vi "KillProcessName.vi"(3 "error in (no error)":errorcluster, 5 "Process Name":string="USBSTOR\\DISK*") -> (0 "error out":errorcluster, 1 "Success":bool=TRUE, 2 "Command Output":string="USBSTOR\\DISK&VEN_KINGSTON&PROD_DT_101_G2&REV_PMAP\\001CC0EC34C7EB8145E3016C&0: Kingston DT 101 G2 USB Device\r\nUSBSTOR\\DISK&VEN_SANDISK&PROD_CRUZER&REV_1.00\\20043411200CF763653E&0: SanDisk Cruzer USB Device\r\n2 matching device(s) found.\r\n")   [LabVIEW 2013]
doc: "This VI can restart a usb device or disconnect first then scan for new device."
panel:
  out "return code":i32
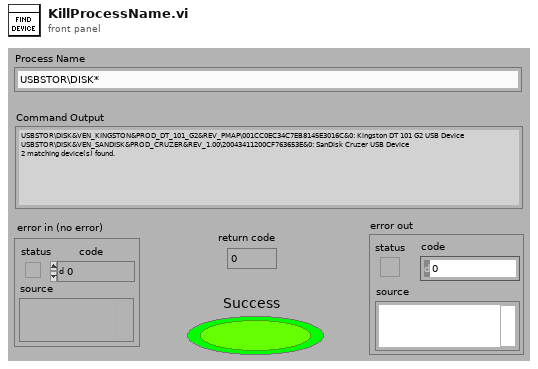
[diagram p1: front panel]
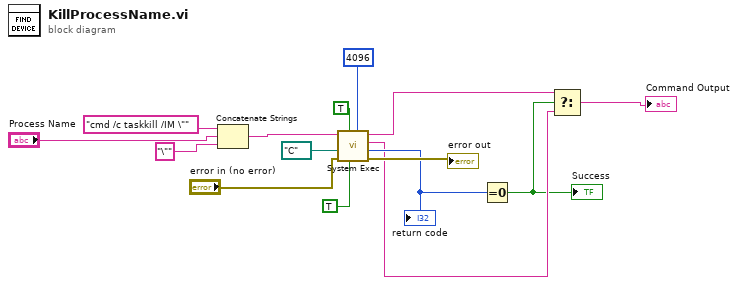
[diagram p0: block diagram]
diagram:
  n1 = Concatenate Strings("cmd /c taskkill /IM \"" ("command line"), "Process Name", "\"" ("string")) -> (w11:string)
  n2 = call <vilib>:"System Exec.vi"("expected output size  (4096)"=u32 4096, "run minimized? (F)"=TRUE, "wait until completion? (T)"=TRUE, "error in (no error)"="error in (no error)", "working directory"=path "C:/", "command line"=w11) -> ("error out"=→"error out":errorcluster, "return code"=w5:i32, "standard error"=w3:string, "standard output"=w4:string)  [unwired: 2 in]
  "return code" <- w5
  n3 = Equal To 0?(x=w5) -> (x = 0?=w2:bool)
  "Success" <- w2
  n4 = Select(t=w4, s=w2, f=w3) -> (s? t:f=→"Command Output":string)
